vi "detect controller.vi"(6 "Network Adapters":bool caption="network adapters (F)", 8 "error in":errorcluster, 11 "controller in":refnum<class "Controller.lvclass">) -> (0 "error out":errorcluster, 3 "controller out":refnum<class "Controller.lvclass">)   [LabVIEW 2013, in "SMI.lvlib" / "Controller.lvclass"]
uses:
  Controller.lvclass
  SysCfg Device/read system session.vi
  SysCfg Device/write system session.vi
  Device/write vendor name.vi
  Device/write product name.vi
  Device/write product ID.vi
  Device/write serial number.vi
  Device/write device class.vi
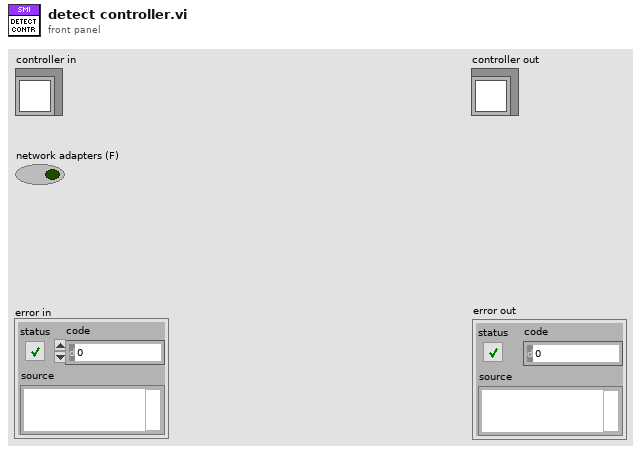
[diagram p1: front panel]
types:
  T1 = typedef "SMI.lvlib/Controller.lvclass/controller information.ctl" = cluster{"system session":refnum<data-value>, "system hardware ref":refnum<data-value>, "vendor name":string, "product name":string, "product ID":u16, "serial number":string, "device information":T2, "primary network adapter":T3, "secondary network adapters":T3[]}
  T2 = typedef "SMI.lvlib/Controller.lvclass/device information.ctl" = cluster{"resource":string, "device class":string, "system start time":timestamp, "current time":timestamp, "time zone":string, "firmware revision":string, "image title":string, "image version":string, "system status":string}
  T3 = typedef "SMI.lvlib/Controller.lvclass/network adapter settings.ctl" = cluster{"IP address":string, "MAC address":string, "IP address request mode":u32, "subnet mask":string, "gateway":string, "DNS server":string, "adapter mode":u32, "adapter type":u32}
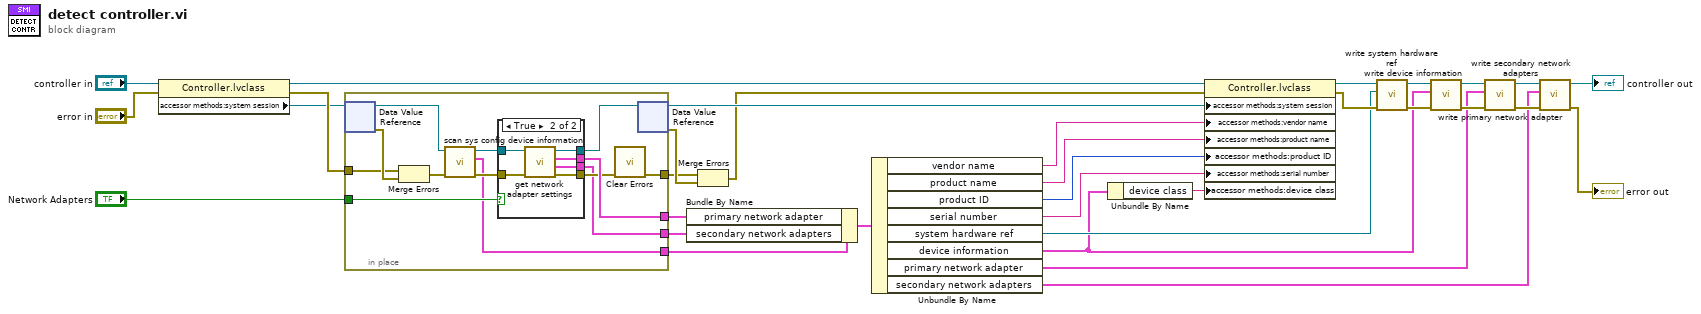
[diagram p0: block diagram]
diagram:
  n1 = property class="Controller.lvclass"(reference="controller in", error in="error in") -> (reference out=w10:refnum<class "Controller.lvclass">, error out=w27:errorcluster, "accessor methods:system session"=w9:refnum<data-value>)
  n2 = in-place {
    in-place-border: "Network Adapters" -> [w46]
    in-place-border: [w43] -> w32
    in-place-border: [w41] -> w31
    in-place-border: [w40] -> w30
    in-place-border: w27 -> [w36]
    in-place-border: [w39] -> w7
    n3 = in-place-dvr #1(w9) -> (w38:refnum<k21>, w37:errorcluster)
    n4 = Merge Errors(w36, w37) -> (w35:errorcluster)
    n5 = call "scan sys config device information.vi"("error in"=w35, "system session in"=w38) -> ("error out"=w44:errorcluster, "controller information"=w41:T1, "system session out"=w45:refnum<k21>)  [unwired: 7 in]
    n6 = case shown="True" w46 {
      tunnel: w45 -> [w48 w54]
      tunnel: w44 -> [w47 w53]
      tunnel: [_ w52] -> w43
      tunnel: [w48 w51] -> w34
      tunnel: [w47 w50] -> w42
      tunnel: [_ w49] -> w40
      frame False {
      }
      frame True {
        n7 = call "get network adapter settings.vi"("error in"=w53, "system session in"=w54) -> ("error out"=w50:errorcluster, "secondary network adapters"=w49:T3[], "primary network adapter"=w52:T3, "system session out"=w51:refnum<k21>)  [unwired: 6 in]
      }
    }
    n8 = call <vilib>:"Clear Errors.vi"("error in (no error)"=w42) -> ("error out"=w39:errorcluster)  [unwired: 6 in]
    n9 = in-place-dvr #1(w34) -> (w5:refnum<data-value>, w8:errorcluster)
  }
  n10 = Bundle By Name(cluster=w31, "primary network adapter"=w32, "secondary network adapters"=w30) -> (w26:T1)
  n11 = Merge Errors(w7, w8) -> (w3:errorcluster)
  n12 = Unbundle By Name(w26) -> ("vendor name"=w6:string, "product name"=w13:string, "product ID"=w12:u16, "serial number"=w11:string, "system hardware ref"=w4:refnum<data-value>, "device information"=w2:T2, "primary network adapter"=w17:T3, "secondary network adapters"=w16:T3[])
  n13 = Unbundle By Name(w2) -> ("device class"=w1:string)
  n14 = property class="Controller.lvclass"(reference=w10, error in=w3, "accessor methods:system session"=w5, "accessor methods:vendor name"=w6, "accessor methods:product name"=w13, "accessor methods:product ID"=w12, "accessor methods:serial number"=w11, "accessor methods:device class"=w1) -> (reference out=w15:refnum<class "Controller.lvclass">, error out=w14:errorcluster)
  n15 = call "write system hardware ref.vi"("error in"=w14, "system hardware ref"=w4, "controller in"=w15) -> ("error out"=w21:errorcluster, "controller out"=w22:refnum<class "Controller.lvclass">)  [unwired: 7 in]
  n16 = call "write device information.vi"("error in"=w21, "device information"=w2, "controller in"=w22) -> ("error out"=w20:errorcluster, "controller out"=w23:refnum<class "Controller.lvclass">)  [unwired: 7 in]
  n17 = call "write primary network adapter.vi"("error in"=w20, "network adapter settings"=w17, "controller in"=w23) -> ("error out"=w24:errorcluster, "controller out"=w25:refnum<class "Controller.lvclass">)  [unwired: 7 in]
  n18 = call "write secondary network adapters.vi"("error in"=w24, "secondary network adapters"=w16, "controller in"=w25) -> ("error out"=→"error out":errorcluster, "controller out"=→"controller out":refnum<class "Controller.lvclass">)  [unwired: 7 in]
